vi "Lab08_Task1_Template.vi"() -> ()   [LabVIEW 2021]
uses:
  <vilib>/userDefined/High Color/IMAQdx.ctl
  <vilib>/vision/driver/NI_Vision_Acquisition_Software.lvlib
panel:
  out "Image":T1(plugin-control)
  in  "Trigger":bool
  in  "Slider":i32(slide)=3 max=9 scale=0.0..9.0
  in  "Stop analysis":bool
  in  "Frames":i32=10
  in  "VideoMode":u32=10
  in  "Session In":T2="cam0"
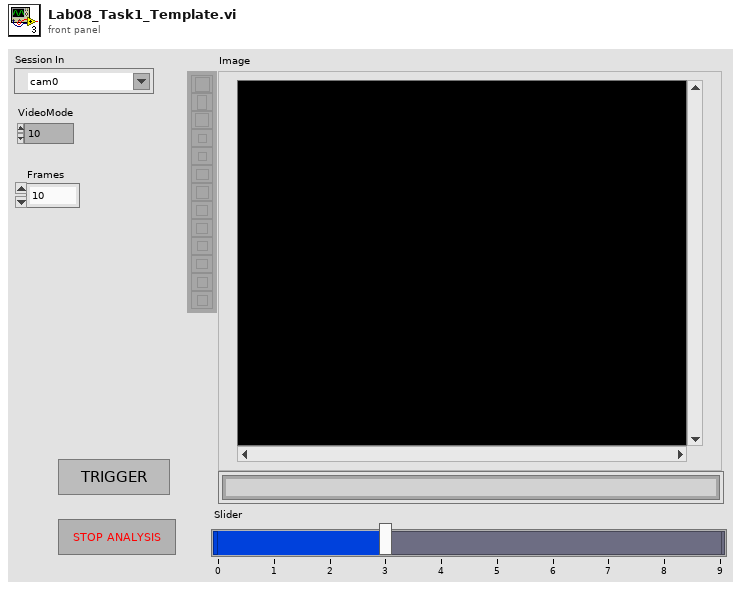
[diagram p1: front panel]
types:
  T1 = typedef "IMAQ Image.ctl" = refnum<image>
  T2 = typedef "IMAQdx.ctl" = refnum<k21>
  T3 = typedef "IMAQ AVI2 Refnum.ctl" = refnum<k20>
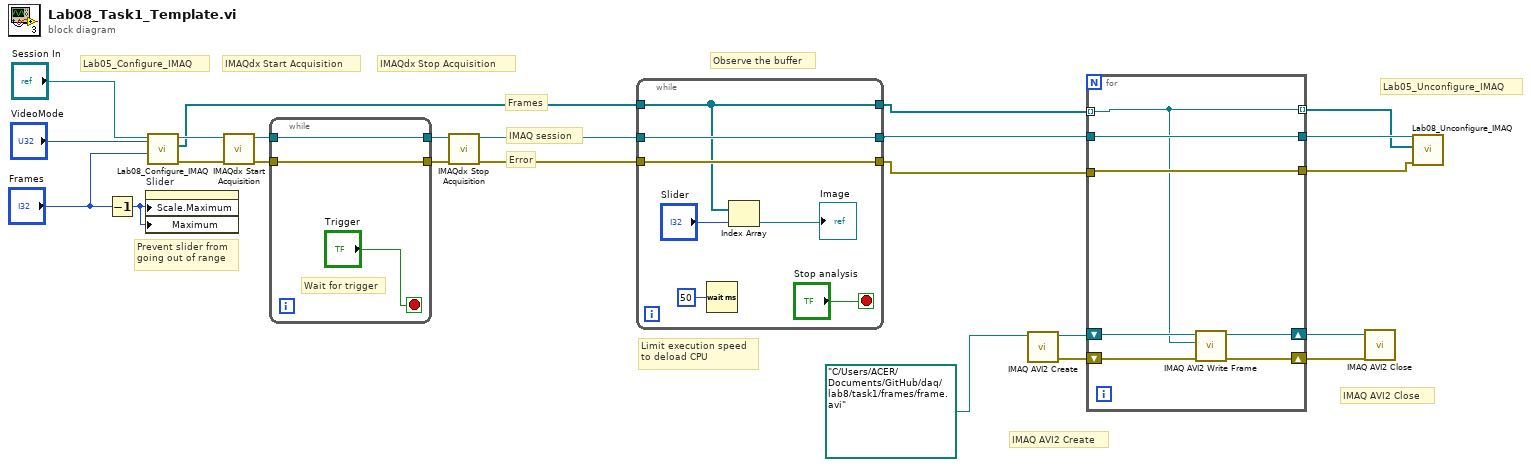
[diagram p0: block diagram]
diagram:
  # "IMAQ AVI2 Create"
  # "IMAQ AVI2 Close"
  # "Limit execution speed\nto deload CPU"
  # "Error"
  # "IMAQ session"
  # "Frames"
  # "Observe the buffer"
  # "Prevent slider from\ngoing out of range"
  # "Lab05_Unconfigure_IMAQ"
  # "Lab05_Configure_IMAQ"
  # "IMAQdx Stop Acquisition"
  # "IMAQdx Start Acquisition"
  n1 = Decrement(x="Frames") -> (x-1=w15:i32)
  n2 = property on="Slider" class="Slide (strict)"("Scale.Maximum"=w15, "Maximum"=w15) -> ()  [unwired: 2 in, 2 out]
  n3 = call "Lab08_Configure_IMAQ.vi"("Frames"="Frames", "VideoMode"="VideoMode", "Session In"="Session In") -> ("error out"=w21:errorcluster, "Images Out"=w14:T1[], "Session Out"=w22:T2)  [unwired: 2 in]
  n4 = call <vilib>:"IMAQdx Start Acquisition.vi"("error in"=w21, "Session In"=w22) -> ("error out"=w19:errorcluster, "Session Out"=w20:T2)  [unwired: 8 out]
  n5 = while {
    tunnel: w20 -> [w26]
    tunnel: w19 -> [w27]
    tunnel: [w27] -> w18
    tunnel: [w26] -> w17
    stop <- "Trigger" stop-if-true
    # "Wait for trigger"
  }
  n6 = call <vilib>:"IMAQdx Stop Acquisition.vi"("error in"=w18, "Session In"=w17) -> ("error out"=w12:errorcluster, "Session Out"=w13:T2)  [unwired: 8 out]
  n7 = while {
    tunnel: w14 -> [w29]
    tunnel: [w29] -> w4
    tunnel: w13 -> [w31]
    tunnel: [w31] -> w5
    tunnel: w12 -> [w30]
    tunnel: [w30] -> w6
    stop <- "Stop analysis" stop-if-true
    n8 = Wait (ms)(milliseconds to wait=u32 50) -> ()  [unwired: 1 out]
    n9 = Index Array "Index Array"(array=w29, index="Slider") -> (element=→"Image":T1)
  }
  n10 = call "IMAQ AVI2 Create"("AVI Path"=path "C:/Users/ACER/Documents/GitHub/daq/lab8/task1/frames/frame.avi") -> ("error out"=w9:errorcluster, "AVI Refnum"=w8:T3)  [unwired: 9 in]
  n11 = for {
    shift-right: [w41] -> w11
    shift-left: w8 -> [w38]
    shift-right: [w40] -> w10
    shift-left: w9 -> [w39]
    tunnel: w6 -> [w37]
    tunnel: w5 -> [w36]
    tunnel: w4 -> [w35] mode=indexing
    tunnel: [w37] -> w3
    tunnel: [w36] -> w2
    tunnel: [w35] -> w1 mode=indexing
    n12 = call "IMAQ AVI2 Write Frame"("error in (no error)"=w39, "Image"=w35, "AVI Refnum"=w38) -> ("error out"=w40:errorcluster, "AVI Refnum (duplicate)"=w41:T3)  [unwired: 6 in, 1 out]
  }
  n13 = call "IMAQ AVI2 Close"("error in (no error)"=w10, "AVI Refnum"=w11) -> ()  [unwired: 9 in, 1 out]
  n14 = call "Lab08_Unconfigure_IMAQ.vi"("error in (no error)"=w3, "Images to dispose"=w1, "IMAQdx session in"=w2) -> ()  [unwired: 8 in, 1 out]
